vi "战舰得分+音乐vi.vi"() -> ()   [LabVIEW 2018]
panel:
  out "敌机是否入侵":bool
  out "得分":dbl
  out "战舰爆炸":picture
  out "血量":dbl
  out "战舰血量":T1 scale=0.0..100.0
  out "敌机爆炸":picture
  in  "敌机数量":dbl
  in  "敌机速度":dbl
  out "敌机":picture
  out "按键":dbl
  out "战舰":T2
  out "激光武器1":T3
  out "激光武器 2":T3
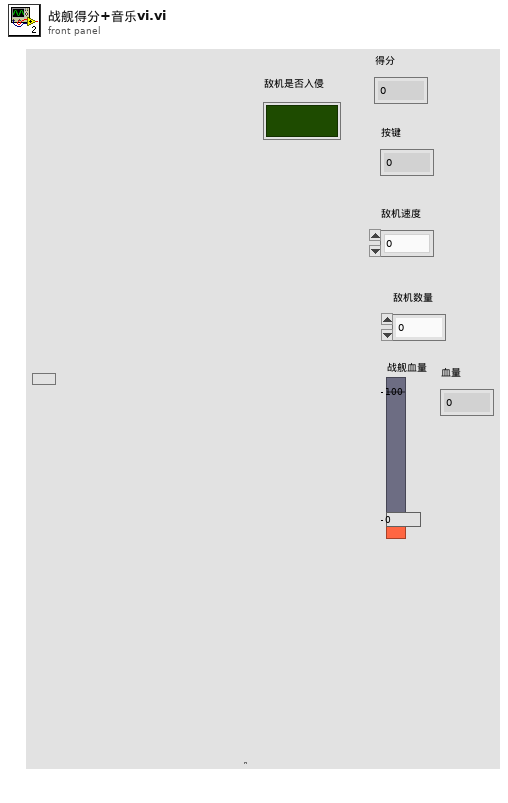
[diagram p1: front panel]
types:
  T1 = typedef "战列巡洋舰_血条.ctl" = dbl
  T2 = typedef "战列巡洋舰.ctl" = picture
  T3 = typedef "战列巡洋舰_激光武器.ctl" = picture
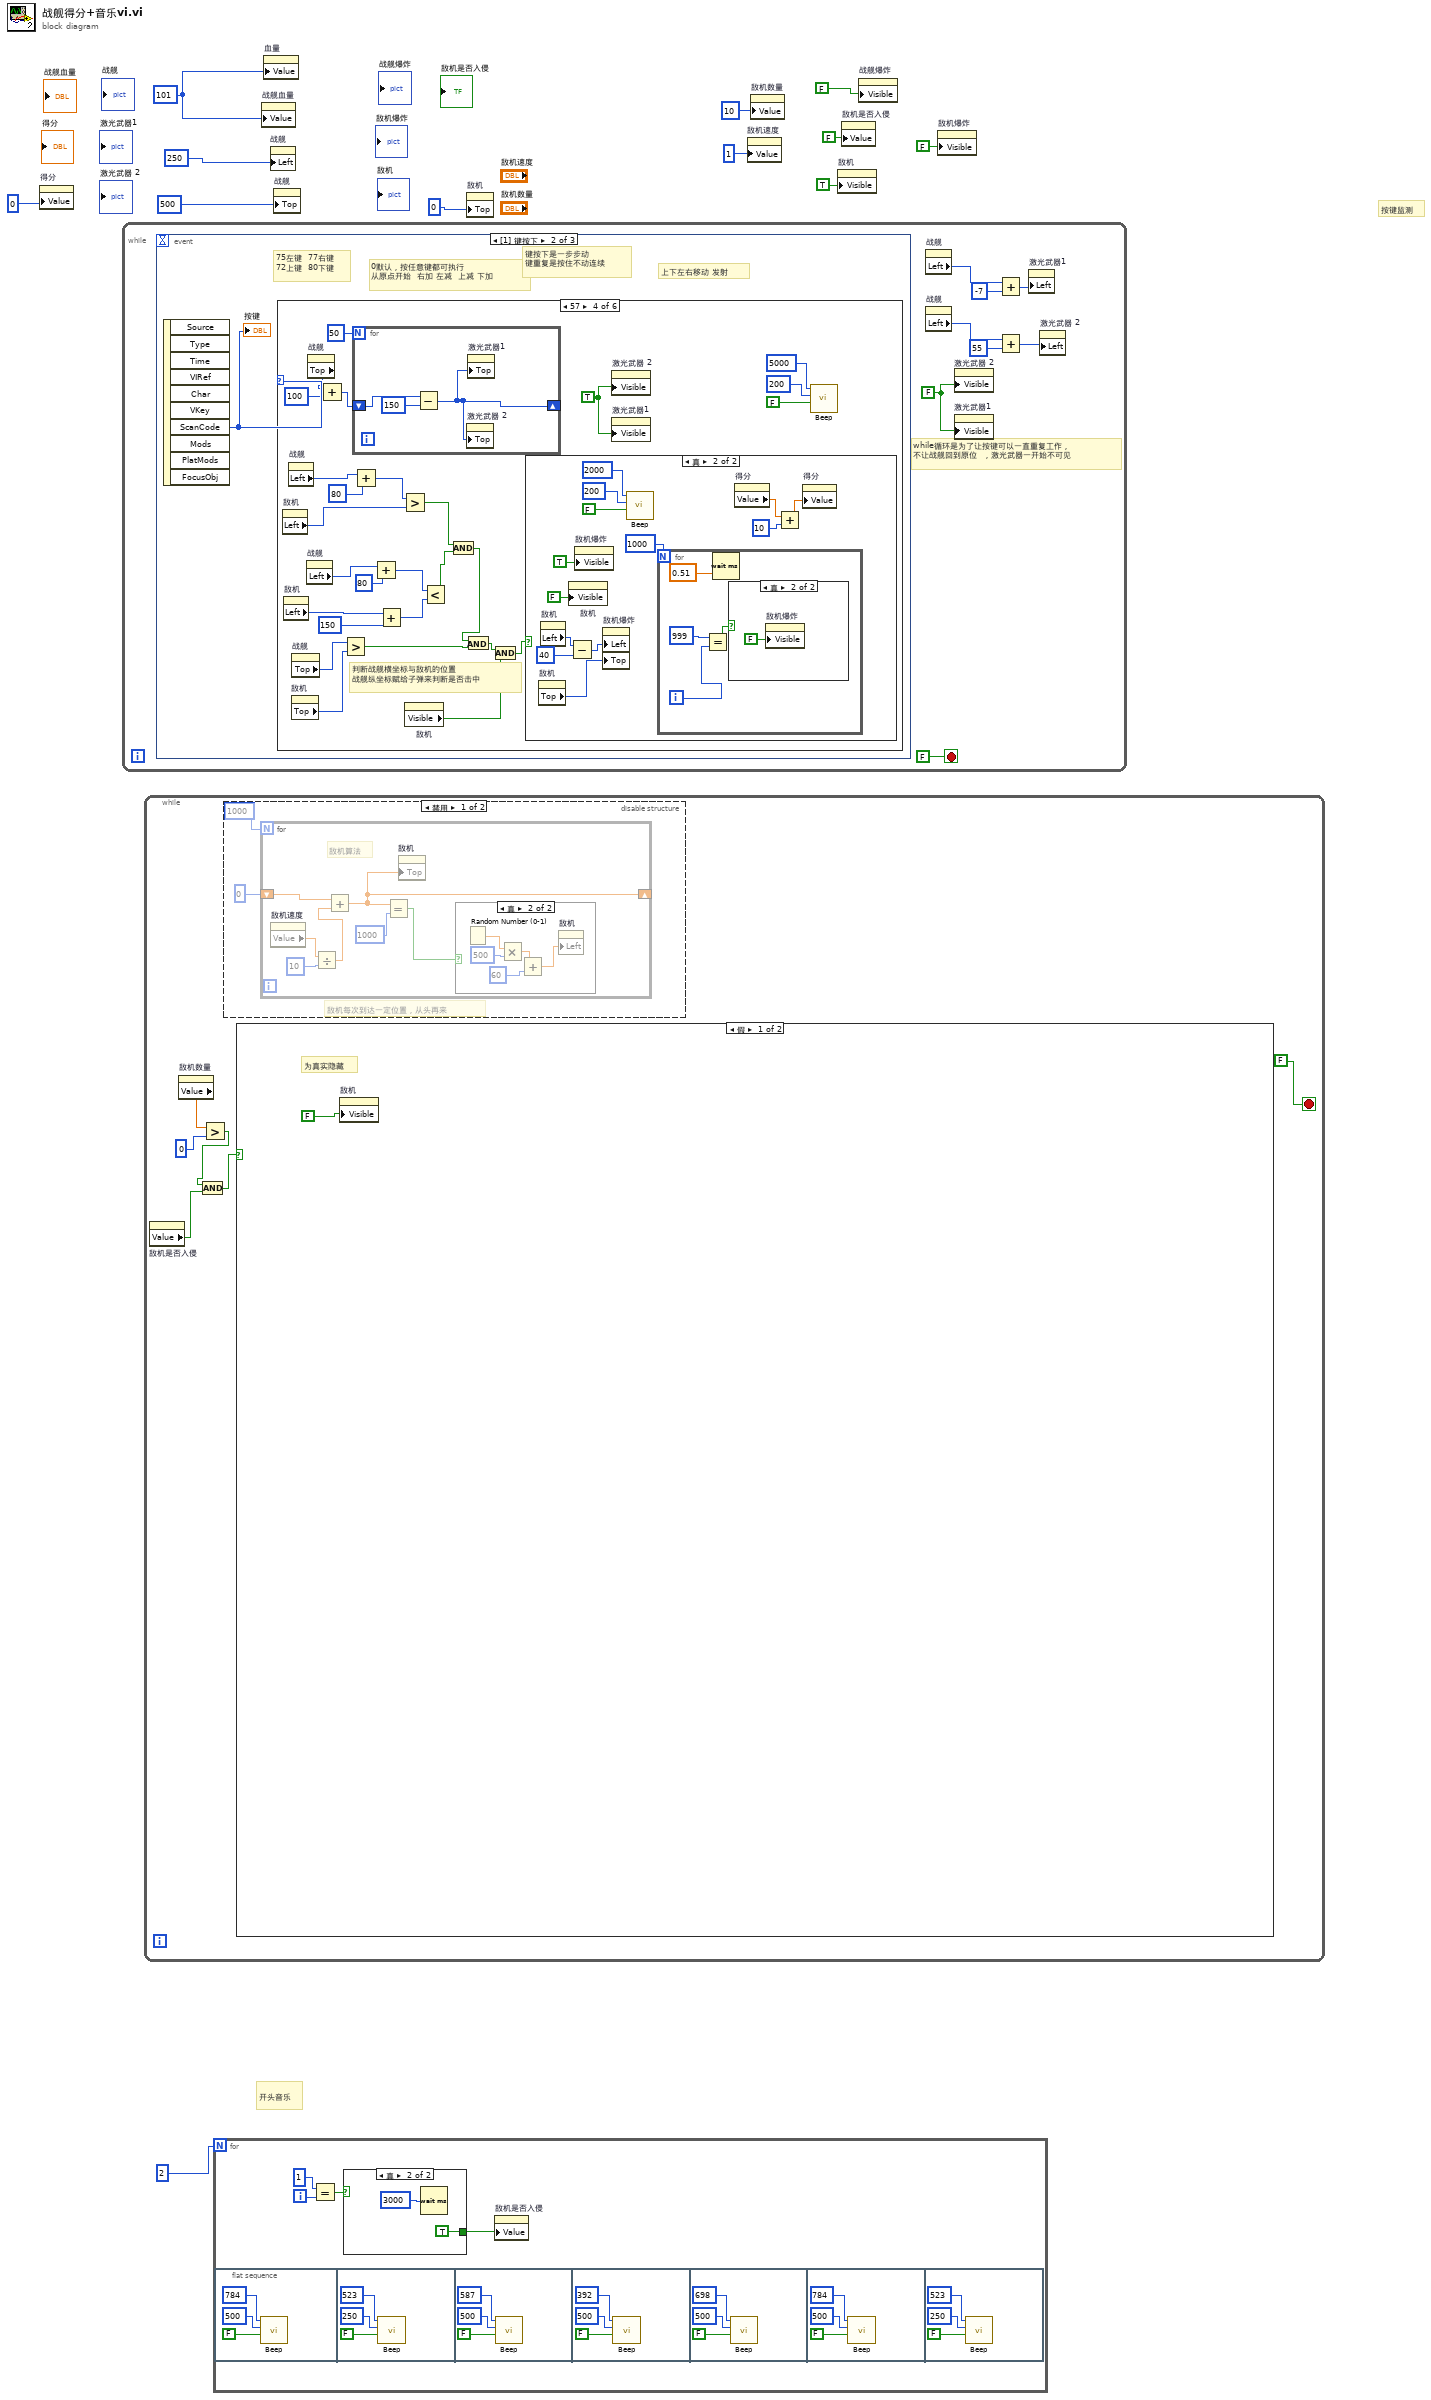
[diagram p0: block diagram]
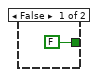
[diagram p2: hidden frame]
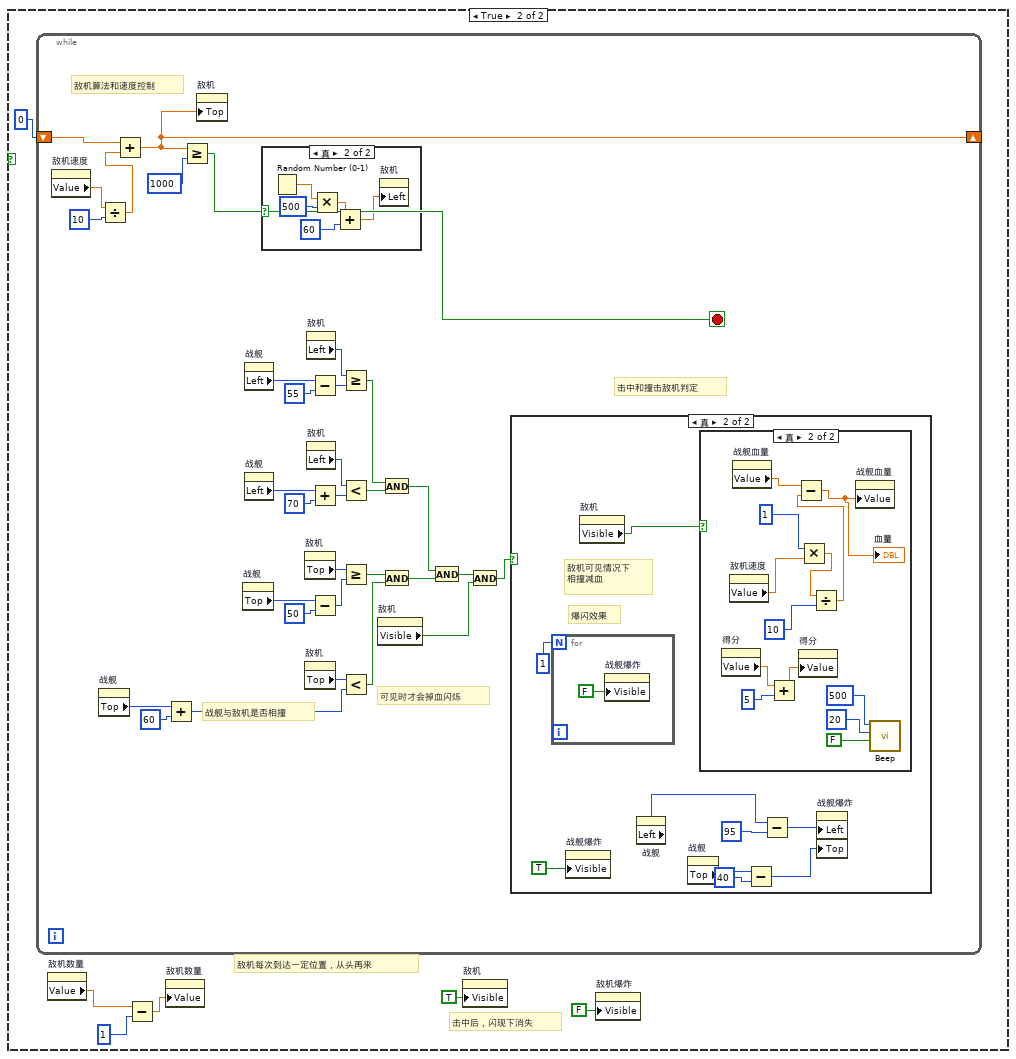
[diagram p3: hidden frame]
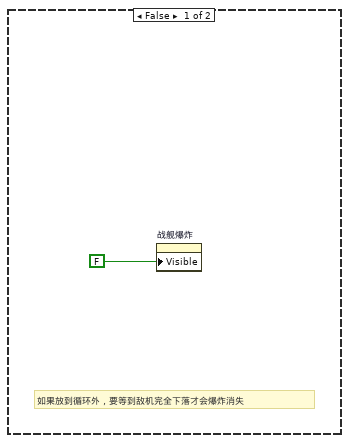
[diagram p4: hidden frame]
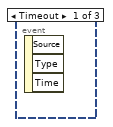
[diagram p9: hidden frame]
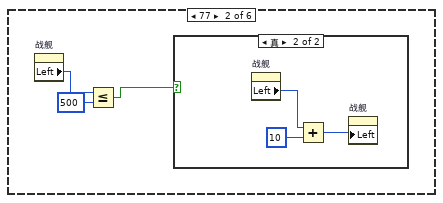
[diagram p11: hidden frame]
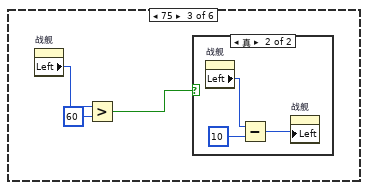
[diagram p13: hidden frame]
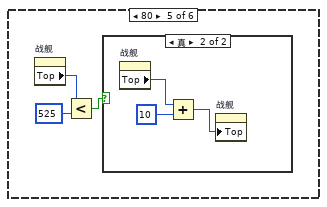
[diagram p17: hidden frame]
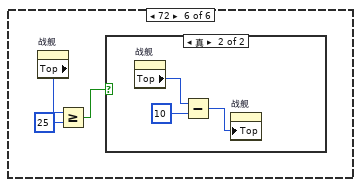
[diagram p19: hidden frame]
diagram:
  w6 = 101
  # "开头音乐"
  # "按键监测"
  n1 = property on="得分" class="DigNum (严格)"("Value"=0) -> ()  [unwired: 2 in, 2 out]
  n2 = while {
    stop <- FALSE stop-if-true
    w13 = FALSE
    # "while循环是为了让按键可以一直重复工作，\n不让战舰回到原位  ，激光武器一开始不可见"
    n3 = event shown="[1] 键按下" {
      selector: _ -> [_ _ _]
      dyn-events: _ -> [_ _ _]
      timeout: _ -> [_ _ _]
      event Timeout {
        n4 = event-data() -> ()  [unwired: 1 in, 3 out]
      }
      event Key Down {
        # "上下左右移动 发射"
        # "键按下是一步步动\n键重复是按住不动连续"
        # "75左键  77右键\n72上键  80下键"
        # "0默认，按任意键都可执行\n从原点开始  右加 左减  上减 下加"
        n5 = event-data() -> ("ScanCode"=w21:i16)  [unwired: 1 in, 9 out]
        "按键" <- w21
        n6 = case shown="57" w21 {
          frame 0, Default {
          }
          frame 77 {
            n7 = property on="战舰" class="Pict (严格)"() -> ("Left"=w24:i32)  [unwired: 2 in, 2 out]
            n8 = Less Or Equal?(x=w24, y=500) -> (x <= y?=w22:bool)
            n9 = case shown="真" w22 {
              frame False {
              }
              frame True {
                n10 = property on="战舰" class="Pict (严格)"() -> ("Left"=w26:i32)  [unwired: 2 in, 2 out]
                n11 = Add(x=w26, y=10) -> (x+y=w27:i32)
                n12 = property on="战舰" class="Pict (严格)"("Left"=w27) -> ()  [unwired: 2 in, 2 out]
              }
            }
          }
          frame 75 {
            n13 = property on="战舰" class="Pict (严格)"() -> ("Left"=w30:i32)  [unwired: 2 in, 2 out]
            n14 = Greater?(x=w30, y=60) -> (0:w28:bool)
            n15 = case shown="真" w28 {
              frame False {
              }
              frame True {
                n16 = property on="战舰" class="Pict (严格)"() -> ("Left"=w32:i32)  [unwired: 2 in, 2 out]
                n17 = Subtract(x=w32, y=10) -> (x-y=w33:i32)
                n18 = property on="战舰" class="Pict (严格)"("Left"=w33) -> ()  [unwired: 2 in, 2 out]
              }
            }
          }
          frame 57 {
            w56 = TRUE
            # "判断战舰横坐标与敌机的位置\n战舰纵坐标赋给子弹来判断是否击中"
            n19 = property on="敌机" class="Pict"() -> ("Left"=w53:i32)  [unwired: 2 in, 2 out]
            n20 = property on="敌机" class="Pict"() -> ("Left"=w46:i32)  [unwired: 2 in, 2 out]
            n21 = property on="战舰" class="Pict (严格)"() -> ("Left"=w55:i32)  [unwired: 2 in, 2 out]
            n22 = property on="敌机" class="Pict"() -> ("Top"=w40:i32)  [unwired: 2 in, 2 out]
            n23 = property on="战舰" class="Pict (严格)"() -> ("Top"=w41:i32)  [unwired: 2 in, 2 out]
            n24 = property on="战舰" class="Pict (严格)"() -> ("Left"=w48:i32)  [unwired: 2 in, 2 out]
            n25 = property on="战舰" class="Pict (严格)"() -> ("Top"=w59:i32)  [unwired: 2 in, 2 out]
            n26 = Add(x=w59, y=100) -> (x+y=w57:i32)
            n27 = Greater?(x=w41, y=w40) -> (0:w42:bool)
            n28 = for {
              N: 50 -> [_]
              shift-right: [w79] -> _
              shift-left: w57 -> [w81]
              n29 = Subtract(x=w81, y=150) -> (x-y=w79:i32)
              n30 = property on="激光武器 2" class="Pict (严格)"("Top"=w79) -> ()  [unwired: 2 in, 2 out]
              n31 = property on="激光武器1" class="Pict (严格)"("Top"=w79) -> ()  [unwired: 2 in, 2 out]
            }
            n32 = Add(x=w55, y=80) -> (x+y=w52:i32)
            n33 = Add(x=w48, y=80) -> (x+y=w50:i32)
            n34 = Add(x=w46, y=150) -> (x+y=w45:i32)
            n35 = Greater?(x=w52, y=w53) -> (0:w51:bool)
            n36 = property on="敌机" class="Pict"() -> ("Visible"=w38:bool)  [unwired: 2 in, 2 out]
            n37 = Less?(x=w50, y=w45) -> (x < y?=w47:bool)
            n38 = And(x=w51, y=w47) -> (x .and. y?=w43:bool)
            n39 = And(x=w43, y=w42) -> (x .and. y?=w39:bool)
            n40 = And(x=w39, y=w38) -> (x .and. y?=w37:bool)
            n41 = case shown="真" w37 {
              frame False {
              }
              frame True {
                n42 = property on="敌机" class="Pict"() -> ("Top"=w71:i32)  [unwired: 2 in, 2 out]
                n43 = property on="敌机" class="Pict"() -> ("Left"=w69:i32)  [unwired: 2 in, 2 out]
                n44 = property on="敌机" class="Pict"("Visible"=FALSE ("可见")) -> ()  [unwired: 2 in, 2 out]
                n45 = Subtract(x=w69, y=40) -> (x-y=w68:i32)
                n46 = property on="敌机爆炸" class="Pict"("Visible"=TRUE ("可见")) -> ()  [unwired: 2 in, 2 out]
                n47 = property on="敌机爆炸" class="Pict"("Left"=w68, "Top"=w71) -> ()  [unwired: 2 in, 2 out]
                n48 = call <vilib>:"Beep.vi"("use system alert? (T)"=FALSE, "duration (msec)"=u32 200, "frequency (Hz)"=u32 2000) -> ()  [unwired: 9 in]
                n49 = for {
                  N: 1000 -> [_]
                  i -> [w76]
                  n50 = Equal?(x=999, y=w76) -> (x = y?=w77:bool)
                  n51 = Wait (ms)(milliseconds to wait=0.51) -> ()  [unwired: 1 out]
                  n52 = case shown="真" w77 {
                    frame False {
                    }
                    frame True {
                      n53 = property on="敌机爆炸" class="Pict"("Visible"=FALSE ("可见")) -> ()  [unwired: 2 in, 2 out]
                    }
                  }
                }
                n54 = property on="得分" class="DigNum (严格)"() -> ("Value"=w66:dbl)  [unwired: 2 in, 2 out]
                n55 = Add(x=w66, y=10) -> (x+y=w64:dbl)
                n56 = property on="得分" class="DigNum (严格)"("Value"=w64) -> ()  [unwired: 2 in, 2 out]
              }
            }
            n57 = property on="激光武器 2" class="Pict (严格)"("Visible"=w56) -> ()  [unwired: 2 in, 2 out]
            n58 = property on="激光武器1" class="Pict (严格)"("Visible"=w56) -> ()  [unwired: 2 in, 2 out]
            n59 = call <vilib>:"Beep.vi"("use system alert? (T)"=FALSE, "duration (msec)"=u32 200, "frequency (Hz)"=u32 5000) -> ()  [unwired: 9 in]
          }
          frame 80 {
            n60 = property on="战舰" class="Pict (严格)"() -> ("Top"=w84:i32)  [unwired: 2 in, 2 out]
            n61 = Less?(x=w84, y=525) -> (x < y?=w82:bool)
            n62 = case shown="真" w82 {
              frame False {
              }
              frame True {
                n63 = property on="战舰" class="Pict (严格)"() -> ("Top"=w86:i32)  [unwired: 2 in, 2 out]
                n64 = Add(x=w86, y=10) -> (x+y=w85:i32)
                n65 = property on="战舰" class="Pict (严格)"("Top"=w85) -> ()  [unwired: 2 in, 2 out]
              }
            }
          }
          frame 72 {
            n66 = property on="战舰" class="Pict (严格)"() -> ("Top"=w90:i32)  [unwired: 2 in, 2 out]
            n67 = Greater Or Equal?(x=w90, y=25) -> (x >= y?=w89:bool)
            n68 = case shown="真" w89 {
              frame False {
              }
              frame True {
                n69 = property on="战舰" class="Pict (严格)"() -> ("Top"=w93:i32)  [unwired: 2 in, 2 out]
                n70 = Subtract(x=w93, y=10) -> (x-y=w92:i32)
                n71 = property on="战舰" class="Pict (严格)"("Top"=w92) -> ()  [unwired: 2 in, 2 out]
              }
            }
          }
        }
      }
      event Key Repeat {
        # "75左键  77右键\n72上键  80下键\n空格 57"
        # "0默认，按任意键都可执行\n从原点开始  右加 左减  上减 下加"
        n72 = event-data() -> ("ScanCode"=w94:i16)  [unwired: 1 in, 9 out]
        n73 = case shown="72" w94 {
          frame 0, Default {
          }
          frame 77 {
            n74 = property on="战舰" class="Pict (严格)"() -> ("Left"=w97:i32)  [unwired: 2 in, 2 out]
            n75 = Less Or Equal?(x=w97, y=500) -> (x <= y?=w96:bool)
            n76 = case shown="真" w96 {
              frame False {
              }
              frame True {
                n77 = property on="战舰" class="Pict (严格)"() -> ("Left"=w99:i32)  [unwired: 2 in, 2 out]
                n78 = Add(x=w99, y=10) -> (x+y=w100:i32)
                n79 = property on="战舰" class="Pict (严格)"("Left"=w100) -> ()  [unwired: 2 in, 2 out]
              }
            }
          }
          frame 75 {
            n80 = property on="战舰" class="Pict (严格)"() -> ("Left"=w103:i32)  [unwired: 2 in, 2 out]
            n81 = Greater Or Equal?(x=w103, y=25) -> (x >= y?=w102:bool)
            n82 = case shown="真" w102 {
              frame False {
              }
              frame True {
                n83 = property on="战舰" class="Pict (严格)"() -> ("Left"=w106:i32)  [unwired: 2 in, 2 out]
                n84 = Subtract(x=w106, y=10) -> (x-y=w105:i32)
                n85 = property on="战舰" class="Pict (严格)"("Left"=w105) -> ()  [unwired: 2 in, 2 out]
              }
            }
          }
          frame 80 {
            n86 = property on="战舰" class="Pict (严格)"() -> ("Top"=w109:i32)  [unwired: 2 in, 2 out]
            n87 = Less Or Equal?(x=w109, y=525) -> (x <= y?=w108:bool)
            n88 = case shown="真" w108 {
              frame False {
              }
              frame True {
                n89 = property on="战舰" class="Pict (严格)"() -> ("Top"=w111:i32)  [unwired: 2 in, 2 out]
                n90 = Add(x=w111, y=10) -> (x+y=w110:i32)
                n91 = property on="战舰" class="Pict (严格)"("Top"=w110) -> ()  [unwired: 2 in, 2 out]
              }
            }
          }
          frame 72 {
            n92 = property on="战舰" class="Pict (严格)"() -> ("Top"=w115:i32)  [unwired: 2 in, 2 out]
            n93 = Greater Or Equal?(x=w115, y=25) -> (x >= y?=w114:bool)
            n94 = case shown="真" w114 {
              frame False {
              }
              frame True {
                n95 = property on="战舰" class="Pict (严格)"() -> ("Top"=w118:i32)  [unwired: 2 in, 2 out]
                n96 = Subtract(x=w118, y=10) -> (x-y=w117:i32)
                n97 = property on="战舰" class="Pict (严格)"("Top"=w117) -> ()  [unwired: 2 in, 2 out]
              }
            }
          }
        }
      }
    }
    n98 = property on="战舰" class="Pict (严格)"() -> ("Left"=w19:i32)  [unwired: 2 in, 2 out]
    n99 = property on="战舰" class="Pict (严格)"() -> ("Left"=w15:i32)  [unwired: 2 in, 2 out]
    n100 = property on="激光武器 2" class="Pict (严格)"("Visible"=w13) -> ()  [unwired: 2 in, 2 out]
    n101 = property on="激光武器1" class="Pict (严格)"("Visible"=w13) -> ()  [unwired: 2 in, 2 out]
    n102 = Add(x=w19, y=-7) -> (x+y=w18:i32)
    n103 = Add(x=w15, y=55) -> (x+y=w14:i32)
    n104 = property on="激光武器1" class="Pict (严格)"("Left"=w18) -> ()  [unwired: 2 in, 2 out]
    n105 = property on="激光武器 2" class="Pict (严格)"("Left"=w14) -> ()  [unwired: 2 in, 2 out]
  }
  n106 = while {
    stop <- FALSE stop-if-true
    n107 = property on="敌机是否入侵" class="Bool (严格)"() -> ("Value"=w121:bool)  [unwired: 2 in, 2 out]
    n108 = property on="敌机数量" class="DigNum (严格)"() -> ("Value"=w123:dbl)  [unwired: 2 in, 2 out]
    n109 = Greater?(x=w123, y=0) -> (0:w120:bool)
    n110 = And(x=w120, y=w121) -> (x .and. y?=w119:bool)
    n111 = disable-structure shown="禁用" {
      frame Disabled {
        # "敌机每次到达一定位置，从头再来"
        n112 = for {
          N: 1000 -> [_]
          shift-right: [w198] -> _
          shift-left: 0 -> [w201]
          # "敌机算法"
          n113 = property on="敌机速度" class="DigNum (严格)"() -> ("Value"=w197:dbl)  [unwired: 2 in, 2 out]
          n114 = Divide(x=w197, y=10) -> (x/y=w196:dbl)
          n115 = Add(x=w201, y=w196) -> (x+y=w198:dbl)
          n116 = Equal?(x=w198, y=1000) -> (x = y?=w199:bool)
          n117 = property on="敌机" class="Pict"("Top"=w198) -> ()  [unwired: 2 in, 2 out]
          n118 = case shown="真" w199 {
            frame False {
            }
            frame True {
              n119 = Random Number (0-1)() -> (number: 0 to 1=w206:dbl)
              n120 = Multiply(x=w206, y=500) -> (x*y=w204:dbl)
              n121 = Add(x=w204, y=60) -> (x+y=w203:dbl)
              n122 = property on="敌机" class="Pict"("Left"=w203) -> ()  [unwired: 2 in, 2 out]
            }
          }
        }
      }
      frame Enabled {
      }
    }
    n123 = case shown="假" w119 {
      frame False {
        # "为真实隐藏"
        n124 = property on="敌机" class="Pict"("Visible"=FALSE ("可见")) -> ()  [unwired: 2 in, 2 out]
      }
      frame True {
        # "击中后，闪现下消失"
        # "敌机每次到达一定位置，从头再来"
        n125 = while {
          shift-right: [w161] -> _
          shift-left: 0 -> [w163]
          stop <- w157 stop-if-true
          # "击中和撞击敌机判定"
          # "可见时才会掉血闪烁"
          # "战舰与敌机是否相撞"
          # "敌机算法和速度控制"
          n126 = property on="敌机速度" class="DigNum (严格)"() -> ("Value"=w160:dbl)  [unwired: 2 in, 2 out]
          n127 = property on="战舰" class="Pict (严格)"() -> ("Top"=w139:i32)  [unwired: 2 in, 2 out]
          n128 = Divide(x=w160, y=10) -> (x/y=w159:dbl)
          n129 = Add(x=w163, y=w159) -> (x+y=w161:dbl)
          n130 = Add(x=w139, y=60) -> (x+y=w141:i32)
          n131 = Greater Or Equal?(x=w161, y=1000) -> (x >= y?=w157:bool)
          n132 = property on="敌机" class="Pict"("Top"=w161) -> ()  [unwired: 2 in, 2 out]
          n133 = property on="战舰" class="Pict (严格)"() -> ("Top"=w145:i32)  [unwired: 2 in, 2 out]
          n134 = property on="战舰" class="Pict (严格)"() -> ("Left"=w155:i32)  [unwired: 2 in, 2 out]
          n135 = property on="战舰" class="Pict (严格)"() -> ("Left"=w149:i32)  [unwired: 2 in, 2 out]
          n136 = case shown="真" w157 {
            frame False {
            }
            frame True {
              n137 = Random Number (0-1)() -> (number: 0 to 1=w192:dbl)
              n138 = Multiply(x=w192, y=500) -> (x*y=w190:dbl)
              n139 = Add(x=w190, y=60) -> (x+y=w189:dbl)
              n140 = property on="敌机" class="Pict"("Left"=w189) -> ()  [unwired: 2 in, 2 out]
            }
          }
          n141 = property on="敌机" class="Pict"() -> ("Top"=w146:i32)  [unwired: 2 in, 2 out]
          n142 = property on="敌机" class="Pict"() -> ("Top"=w138:i32)  [unwired: 2 in, 2 out]
          n143 = property on="敌机" class="Pict"() -> ("Left"=w156:i32)  [unwired: 2 in, 2 out]
          n144 = property on="敌机" class="Pict"() -> ("Left"=w151:i32)  [unwired: 2 in, 2 out]
          n145 = Subtract(x=w155, y=55) -> (x-y=w154:i32)
          n146 = Add(x=w149, y=70) -> (x+y=w148:i32)
          n147 = Subtract(x=w145, y=50) -> (x-y=w143:i32)
          n148 = Greater Or Equal?(x=w156, y=w154) -> (x >= y?=w152:bool)
          n149 = Less?(x=w151, y=w148) -> (x < y?=w147:bool)
          n150 = Greater Or Equal?(x=w146, y=w143) -> (x >= y?=w137:bool)
          n151 = Less?(x=w138, y=w141) -> (x < y?=w136:bool)
          n152 = property on="敌机" class="Pict"() -> ("Visible"=w133:bool)  [unwired: 2 in, 2 out]
          n153 = And(x=w152, y=w147) -> (x .and. y?=w142:bool)
          n154 = And(x=w137, y=w136) -> (x .and. y?=w135:bool)
          n155 = And(x=w142, y=w135) -> (x .and. y?=w134:bool)
          n156 = And(x=w134, y=w133) -> (x .and. y?=w132:bool)
          n157 = case shown="真" w132 {
            frame False {
              # "如果放到循环外，要等到敌机完全下落才会爆炸消失"
              n158 = property on="战舰爆炸" class="Pict"("Visible"=FALSE ("可见")) -> ()  [unwired: 2 in, 2 out]
            }
            frame True {
              # "爆闪效果"
              # "敌机可见情况下\n相撞减血"
              n159 = for {
                N: 1 -> [_]
                n160 = property on="战舰爆炸" class="Pict"("Visible"=FALSE ("可见")) -> ()  [unwired: 2 in, 2 out]
              }
              n161 = property on="战舰爆炸" class="Pict"("Visible"=TRUE ("可见")) -> ()  [unwired: 2 in, 2 out]
              n162 = property on="敌机" class="Pict"() -> ("Visible"=w173:bool)  [unwired: 2 in, 2 out]
              n163 = property on="战舰" class="Pict (严格)"() -> ("Left"=w171:i32)  [unwired: 2 in, 2 out]
              n164 = property on="战舰" class="Pict (严格)"() -> ("Top"=w168:i32)  [unwired: 2 in, 2 out]
              n165 = case shown="真" w173 {
                frame False {
                }
                frame True {
                  n166 = property on="得分" class="DigNum (严格)"() -> ("Value"=w180:dbl)  [unwired: 2 in, 2 out]
                  n167 = property on="敌机速度" class="DigNum (严格)"() -> ("Value"=w186:dbl)  [unwired: 2 in, 2 out]
                  n168 = property on="战舰血量" class="Slide (严格)"() -> ("Value"=w187:T1)  [unwired: 2 in, 2 out]
                  n169 = Add(x=w180, y=5) -> (x+y=w179:dbl)
                  n170 = Multiply(x=1, y=w186) -> (x*y=w185:dbl)
                  n171 = property on="得分" class="DigNum (严格)"("Value"=w179) -> ()  [unwired: 2 in, 2 out]
                  n172 = Divide(x=w185, y=10) -> (x/y=w182:dbl)
                  n173 = Subtract(x=w187, y=w182) -> (x-y=w181:T1)
                  "血量" <- w181
                  n174 = property on="战舰血量" class="Slide (严格)"("Value"=w181) -> ()  [unwired: 2 in, 2 out]
                  n175 = call <vilib>:"Beep.vi"("use system alert? (T)"=FALSE, "duration (msec)"=u32 20, "frequency (Hz)"=u32 500) -> ()  [unwired: 9 in]
                }
              }
              n176 = Subtract(x=w168, y=40) -> (x-y=w166:i32)
              n177 = Subtract(x=w171, y=95) -> (x-y=w169:i32)
              n178 = property on="战舰爆炸" class="Pict"("Left"=w169, "Top"=w166) -> ()  [unwired: 2 in, 2 out]
            }
          }
        }
        n179 = property on="敌机数量" class="DigNum (严格)"() -> ("Value"=w129:dbl)  [unwired: 2 in, 2 out]
        n180 = Subtract(x=w129, y=1) -> (x-y=w130:dbl)
        n181 = property on="敌机数量" class="DigNum (严格)"("Value"=w130) -> ()  [unwired: 2 in, 2 out]
        n182 = property on="敌机" class="Pict"("Visible"=TRUE ("可见")) -> ()  [unwired: 2 in, 2 out]
        n183 = property on="敌机爆炸" class="Pict"("Visible"=FALSE ("可见")) -> ()  [unwired: 2 in, 2 out]
      }
    }
  }
  n184 = for {
    N: 2 -> [_]
    i -> [w208]
    n185 = flat-sequence {
      frame #0 {
        n186 = call <vilib>:"Beep.vi"("use system alert? (T)"=FALSE, "duration (msec)"=500, "frequency (Hz)"=784) -> ()  [unwired: 9 in]
      }
      frame #1 {
        n187 = call <vilib>:"Beep.vi"("use system alert? (T)"=FALSE, "duration (msec)"=250, "frequency (Hz)"=523) -> ()  [unwired: 9 in]
      }
      frame #2 {
        n188 = call <vilib>:"Beep.vi"("use system alert? (T)"=FALSE, "duration (msec)"=500, "frequency (Hz)"=587) -> ()  [unwired: 9 in]
      }
      frame #3 {
        n189 = call <vilib>:"Beep.vi"("use system alert? (T)"=FALSE, "duration (msec)"=500, "frequency (Hz)"=392) -> ()  [unwired: 9 in]
      }
      frame #4 {
        n190 = call <vilib>:"Beep.vi"("use system alert? (T)"=FALSE, "duration (msec)"=500, "frequency (Hz)"=698) -> ()  [unwired: 9 in]
      }
      frame #5 {
        n191 = call <vilib>:"Beep.vi"("use system alert? (T)"=FALSE, "duration (msec)"=500, "frequency (Hz)"=784) -> ()  [unwired: 9 in]
      }
      frame #6 {
        n192 = call <vilib>:"Beep.vi"("use system alert? (T)"=FALSE, "duration (msec)"=250, "frequency (Hz)"=523) -> ()  [unwired: 9 in]
      }
    }
    n193 = Equal?(x=1, y=w208) -> (x = y?=w210:bool)
    n194 = case shown="真" w210 {
      tunnel: [FALSE ("敌机是否入侵") TRUE ("敌机是否入侵")] -> w207
      frame False {
      }
      frame True {
        n195 = Wait (ms)(milliseconds to wait=u32 3000 ("等待时间（毫秒）")) -> ()  [unwired: 1 out]
      }
    }
    n196 = property on="敌机是否入侵" class="Bool (严格)"("Value"=w207) -> ()  [unwired: 2 in, 2 out]
  }
  n197 = property on="战舰血量" class="Slide (严格)"("Value"=w6) -> ()  [unwired: 2 in, 2 out]
  n198 = property on="血量" class="DigNum (严格)"("Value"=w6) -> ()  [unwired: 2 in, 2 out]
  n199 = property on="战舰" class="Pict (严格)"("Left"=250 ("位置:居左")) -> ()  [unwired: 2 in, 2 out]
  n200 = property on="战舰" class="Pict (严格)"("Top"=500 ("位置:置顶")) -> ()  [unwired: 2 in, 2 out]
  n201 = property on="敌机" class="Pict"("Top"=0) -> ()  [unwired: 2 in, 2 out]
  n202 = property on="敌机速度" class="DigNum (严格)"("Value"=1) -> ()  [unwired: 2 in, 2 out]
  n203 = property on="敌机数量" class="DigNum (严格)"("Value"=10) -> ()  [unwired: 2 in, 2 out]
  n204 = property on="敌机" class="Pict"("Visible"=TRUE ("可见")) -> ()  [unwired: 2 in, 2 out]
  n205 = property on="敌机是否入侵" class="Bool (严格)"("Value"=FALSE ("敌机是否入侵")) -> ()  [unwired: 2 in, 2 out]
  n206 = property on="战舰爆炸" class="Pict"("Visible"=FALSE ("可见")) -> ()  [unwired: 2 in, 2 out]
  n207 = property on="敌机爆炸" class="Pict"("Visible"=FALSE ("可见")) -> ()  [unwired: 2 in, 2 out]
